vi "GA_Fitness.vi"(8 "line_y (500, 20)":dbl[][](array[numeric]), 9 "line_x (500, 20)":dbl[][](array[numeric])) -> (0 "fitness(500)_1":dbl[](array[numeric]), 2 "total_distance(500)":dbl[](array[numeric]), 3 "fitness(500)":dbl[](array[numeric]))   [LabVIEW 2018]
uses:
  GA_Global.vi
panel:
  in  "Numeric 3":i32
  out "Numeric":i32
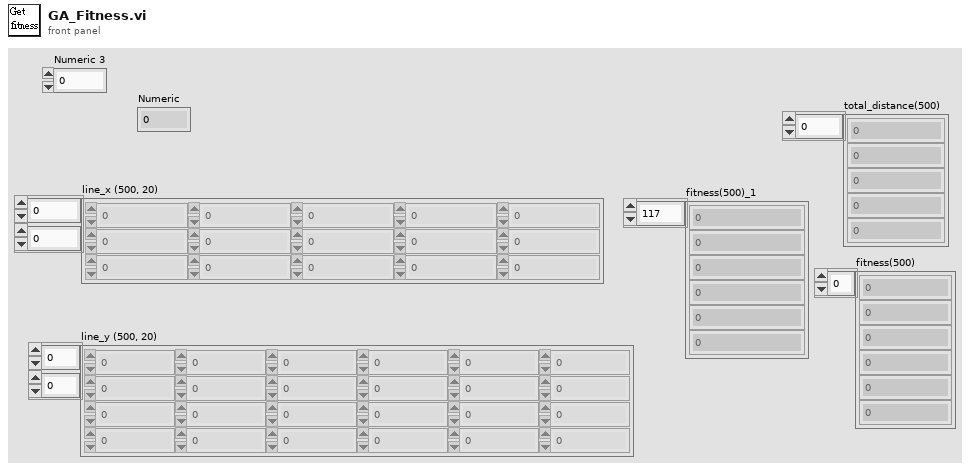
[diagram p1: front panel]
types:
  T1 = typedef "GA_parameter.ctl" = cluster{"N_CITIES":i32, "POP_SIZE":i32, "N_GENERATIONS":i32, "CROSS_RATE":dbl, "MUTATE_RATE":dbl}
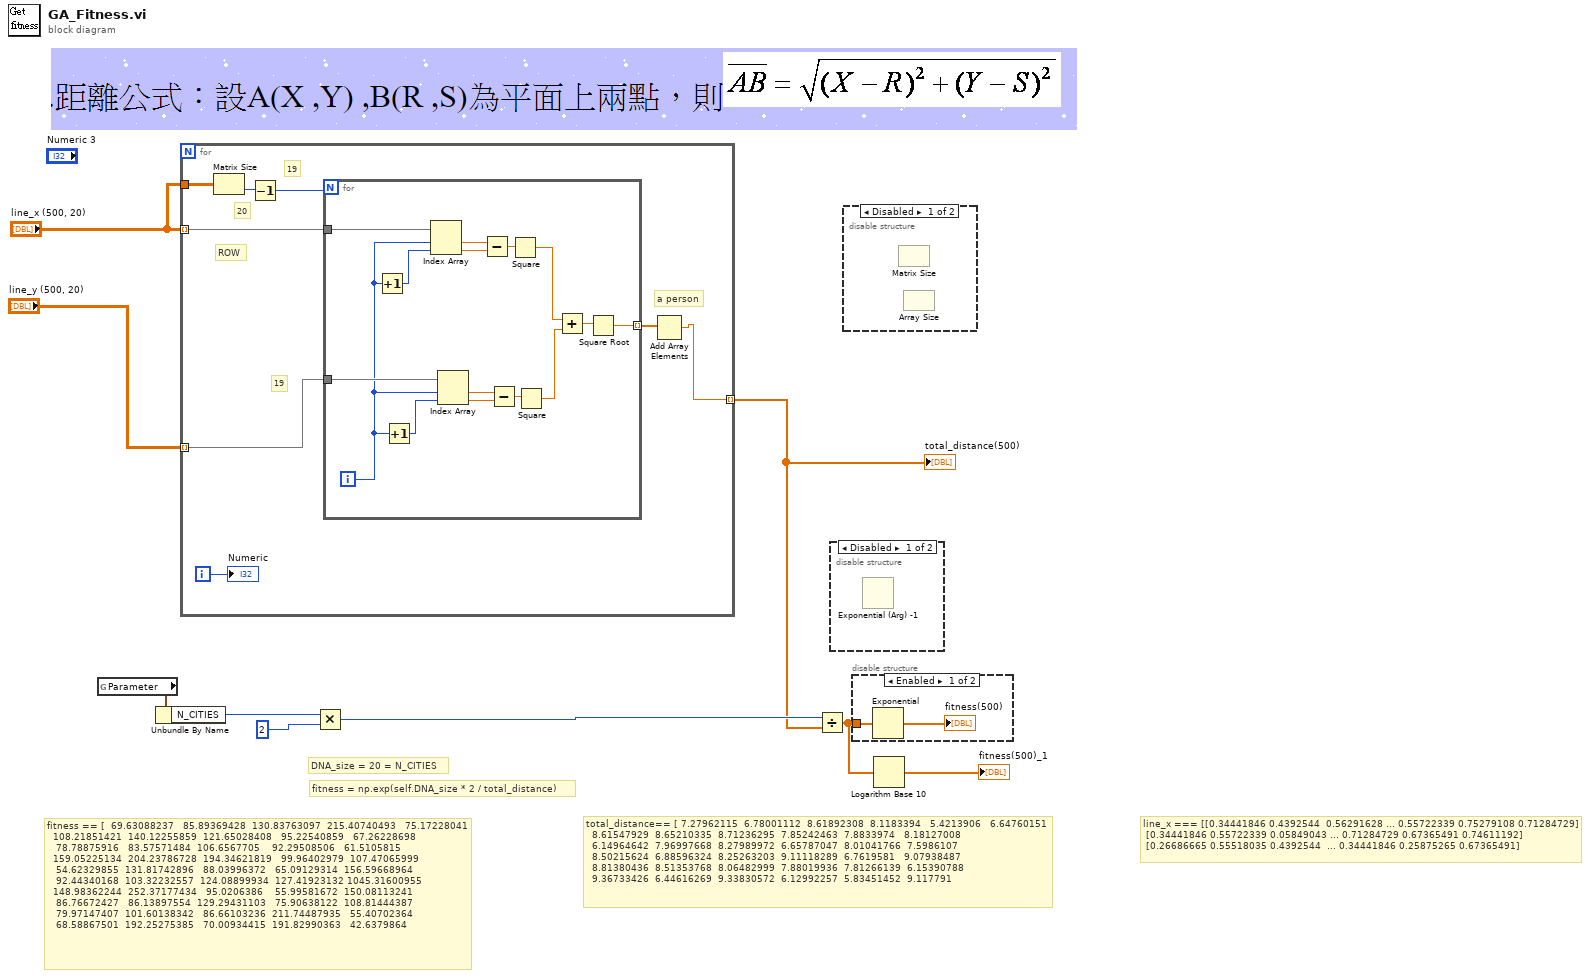
[diagram p0: block diagram]
diagram:
  # "line_x === [[0.34441846 0.4392544  0.56291628 ... 0.55722339 0.75279108 0.71284729]\n [0.34441846 0.55722339 0.05849043 ... 0.71284729 0.67365491 0.74611192]\n [0.26686665 0.55518035 0.4392544  ... 0.34441846 0.25875265 0.67365491]"
  # "total_distance== [ 7.27962115  6.78001112  8.61892308  8.1183394   5.4213906   6.64760151\n  8.61547929  8.65210335  8.71236295  7.85242463  7.8833974   8.18127008\n  6.14964642  7.96997668  8.27989972  6.65787047  8.01041766  7.5986107\n  8.50215624  6.88596324  8.25263203  9.11118289  6.7619581   9.07938487\n  8.81380436  8.51353768  8.06482999  7.88019936  7.81266139  6.15390788\n  9.36733426  6.44616269  9.33830572  6.12992257  5.83451452  9.117791"
  # "fitness == [  69.63088237   85.89369428  130.83763097  215.40740493   75.17228041\n  108.21851421  140.12255859  121.65028408   95.22540859   67.26228698\n   78.78875916   83.57571484  106.6567705    92.29508506   61.5105815\n  159.05225134  204.23786728  194.34621819   99.96402979  107.47065999\n   54.62329855  131.81742896   88.03996372   65.09129314  156.59668964\n   92.44340168  103.32232557  124.08899934  127.41923132 1045.31600955\n  148.98362244  252.37177434   95.0206386    55.99581672  150.08113241\n   86.76672427   86.13897554  129.29431103   75.90638122  108.81444387\n   79.97147407  101.60138342   86.66103236  211.74487935   55.40702364\n   68.58867501  192.25275385   70.00934415  191.82990363   42.6379864"
  # "DNA_size = 20 = N_CITIES"
  # "fitness = np.exp(self.DNA_size * 2 / total_distance)"
  n1 = global read "GA_Global.vi" "Parameter"() -> (w9:T1)
  n2 = Unbundle By Name(w9) -> ("N_CITIES"=w8:i32)
  n3 = for {
    tunnel: "line_x (500, 20)" -> [w15] mode=indexing
    tunnel: "line_x (500, 20)" -> [w13]
    tunnel: "line_y (500, 20)" -> [w12] mode=indexing
    tunnel: [w10] -> w1 mode=indexing
    i -> [w14]
    # "a person"
    # "ROW"
    # "19"
    # "19"
    # "20"
    n4 = Matrix Size(0:w13) -> (2:w17:i32)  [unwired: 1 out]
    n5 = Decrement(x=w17) -> (x-1=w16:i32)
    n6 = for {
      N: w16 -> [_]
      tunnel: w15 -> [w32]
      tunnel: w12 -> [w26]
      tunnel: [w18] -> w11 mode=indexing
      i -> [w25]
      n7 = Increment(x=w25) -> (x+1=w31:i32)
      n8 = Increment(x=w25) -> (x+1=w27:i32)
      n9 = Index Array(array=w32, index #1=w25, index #2=w31) -> (element #1=w29:dbl, element #2=w30:dbl)
      n10 = Index Array(array=w26, index #1=w25, index #2=w27) -> (element #1=w24:dbl, element #2=w23:dbl)
      n11 = Subtract(x=w29, y=w30) -> (x-y=w28:dbl)
      n12 = Subtract(x=w24, y=w23) -> (x-y=w22:dbl)
      n13 = Square(x=w28) -> (x^2=w21:dbl)
      n14 = Square(x=w22) -> (x^2=w20:dbl)
      n15 = Add(x=w21, y=w20) -> (x+y=w19:dbl)
      n16 = Square Root(x=w19) -> (sqrt(x)=w18:dbl)
    }
    n17 = Add Array Elements(numeric array=w11) -> (sum=w10:dbl)
    "Numeric" <- w14
  }
  "total_distance(500)" <- w1
  n18 = Multiply(x=w8, y=2) -> (x*y=w6:i32)
  n19 = Divide(x=w6, y=w1) -> (x/y=w4:dbl[])
  n20 = disable-structure shown="Disabled" {
    frame Disabled {
      n21 = Exponential (Arg) -1() -> ()  [unwired: 1 in, 1 out]
    }
    frame Enabled {
    }
  }
  n22 = disable-structure shown="Disabled" {
    frame Disabled {
      n23 = Matrix Size() -> ()  [unwired: 1 in, 2 out]
      n24 = Array Size() -> ()  [unwired: 1 in, 1 out]
    }
    frame Enabled {
    }
  }
  n25 = disable-structure shown="Enabled" {
    disable-tunnel: w4 -> [w33 _]
    frame Enabled {
      n26 = Exponential(1:w33) -> (0:→"fitness(500)":dbl[])
    }
    frame Disabled {
    }
  }
  n27 = Logarithm Base 10(1:w4) -> (0:→"fitness(500)_1":dbl[])
